vi "write_ui_plot_references.vi"(8 "error in (no error)":errorcluster, 10 "plot_references":T1, 11 "panel in":refnum<class "panel.lvclass">) -> (0 "error out":errorcluster, 3 "panel out":refnum<class "panel.lvclass">)   [LabVIEW 2015, in "panel.lvclass"]
uses:
  panel.lvclass
  front_panel_class/ui_plot_references.ctl
  panel.lvclass/panel.ctl
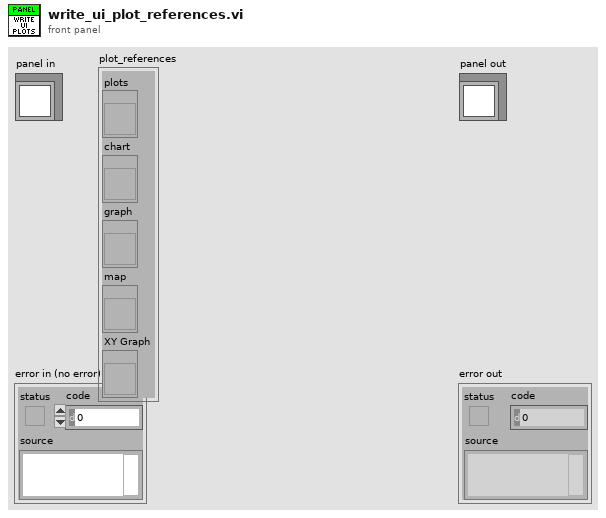
[diagram p1: front panel]
types:
  T1 = typedef "ui_plot_references.ctl" = cluster{"plots":refnum<vi>, "chart":refnum<vi>, "graph":refnum<vi>, "map":refnum<vi>, "XY Graph":refnum<vi>}
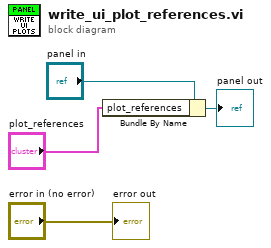
[diagram p0: block diagram]
diagram:
  n1 = Bundle By Name(cluster="panel in", "plot_references"="plot_references") -> (→"panel out":refnum<class "panel.lvclass">)
  "error out" <- "error in (no error)"
